vi "Area.vi"(8 "error in (no error)":errorcluster, 11 "Shape in":refnum<class "Shape.lvclass">) -> (0 "error out":errorcluster, 2 "rect":T1, 3 "Shape out":refnum<class "Shape.lvclass">)   [LabVIEW 2021, in "Picture2D.lvlib" / "Shape.lvclass"]
uses:
  Shape.lvclass
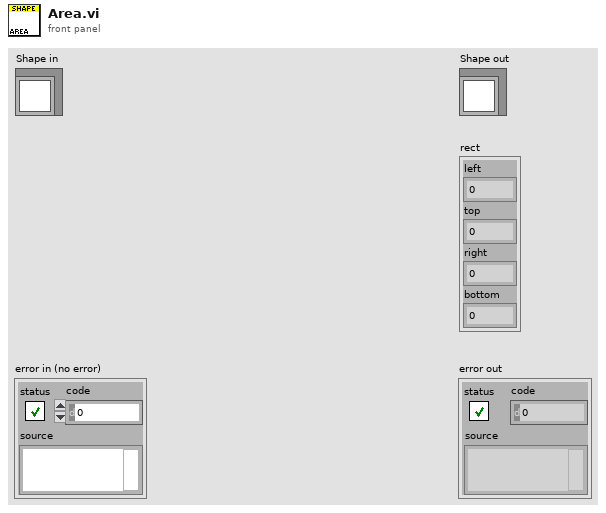
[diagram p1: front panel]
types:
  T1 = cluster{"left":i16, "top":i16, "right":i16, "bottom":i16}
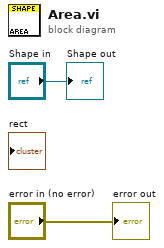
[diagram p0: block diagram]
diagram:
  "error out" <- "error in (no error)"
  "Shape out" <- "Shape in"
